vi "TileWindows.vi"(6 "Front Panel Window:Panel Bounds":T1={"Left"=0, "Top"=20, "Right"=1400, "Bottom"=1400}, 8 "error in (no error)":errorcluster, 10 "Vertical?":bool, 11 "hWnd":i32) -> (0 "error out":errorcluster)   [LabVIEW 2025, in "Test Unit.lvlib"]
uses:
  Test Unit.lvlib
  user32.dll
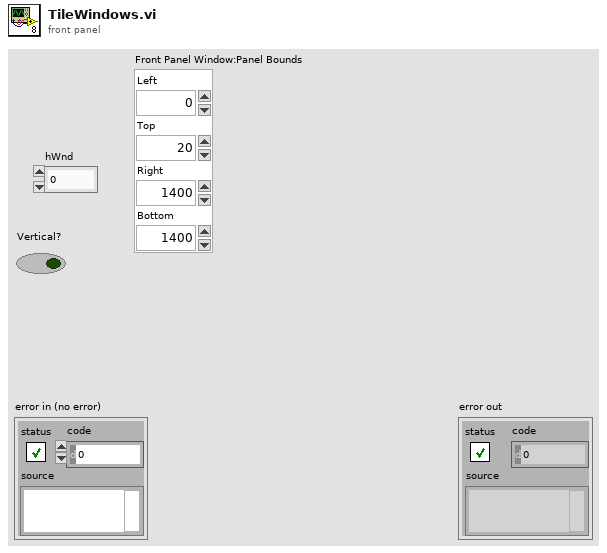
[diagram p1: front panel]
types:
  T1 = cluster{"Left":i32, "Top":i32, "Right":i32, "Bottom":i32}
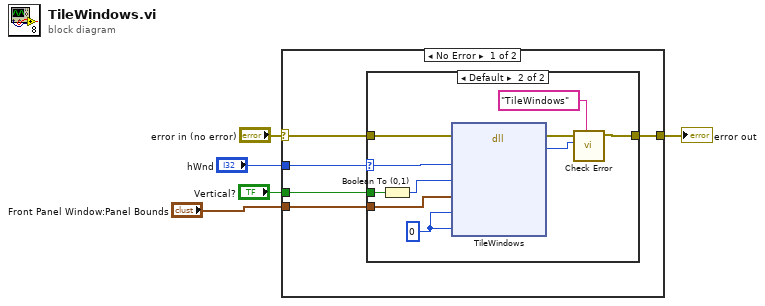
[diagram p0: block diagram]
diagram:
  n1 = case shown="No Error" "error in (no error)" {
    selector: "error in (no error)" -> [w10 w22]
    tunnel: [w9 w22] -> w4
    tunnel: "Vertical?" -> [w8 _]
    tunnel: "hWnd" -> [w7 _]
    tunnel: "Front Panel Window:Panel Bounds" -> [w6 _]
    frame No Error {
      n2 = case shown="Default" w7 {
        selector: w7 -> [_ w19]
        tunnel: w10 -> [w11 w20]
        tunnel: [w11 w13] -> w9
        tunnel: w8 -> [_ w17]
        tunnel: w6 -> [_ w16]
        frame 0 {
        }
        frame Default {
          w21 = u32 0 ("wHow")
          n3 = Boolean To (0,1)(Boolean=w17) -> (0, 1=w18:i16)
          n4 = dll-call lib="user32.dll" fn="TileWindows"(error in=w20, "hwndParent"=w19, "wHow"=w18, "rect"=w16, "cKids"=w21, "lpKids"=w21) -> (error out=w15:errorcluster, "return type"=w14:u32)  [unwired: 7 in, 1 out]
          n5 = call "Check Error.vi"("Description"="TileWindows" ("Error Action"), "Return Code"=w14, "error in (no error)"=w15) -> ("error out"=w13:errorcluster)  [unwired: 8 in]
        }
      }
    }
    frame Error {
    }
  }
  "error out" <- w4
